vi "NaMCU_configure.vi"() -> ()   [LabVIEW 2016]
uses:
  Instrument drivers/Arduino/ctls_and_globals/Arduino tx msg cluster.ctl
panel:
  in  "DIO 1 mode":u8(ring)=1 items=["Input", "Output"]
  in  "DIO 0 mode":u8(ring)=1 items=["Input", "Output"]
  in  "T1 offset (deg C)":dbl
  in  "T0 offset (deg C)":dbl
  in  "P_atmos offset (Pa)":dbl
  in  "Port":refnum<visa-resource-name>
  in  "Get / Set":u8(ring) items=["Get", "Set"]
  in  "Apply pressure corrections":bool=TRUE
  in  "Tube_D (mm)":dbl=1.0
  in  "Tube_L (mm)":dbl
  out "Read-back":string
  in  "dP offset (Pa)":dbl
  out "Status comment":string
  in  "Address":u8=1
  # "Use this vi to configure the NaMCU pressure transducer node\nThese settings are retained in EEPROM and recalled on power-up."
  # "PN 17/01/2017"
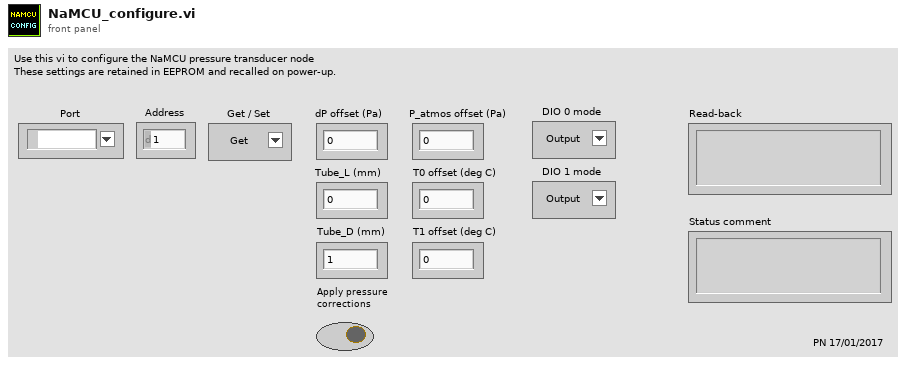
[diagram p1: front panel]
types:
  T1 = typedef "Arduino tx msg cluster.ctl" = cluster{"dest":u8, "A/D/C/I":string, "R/W":string, "chan":u8, "val (float)":sgl}
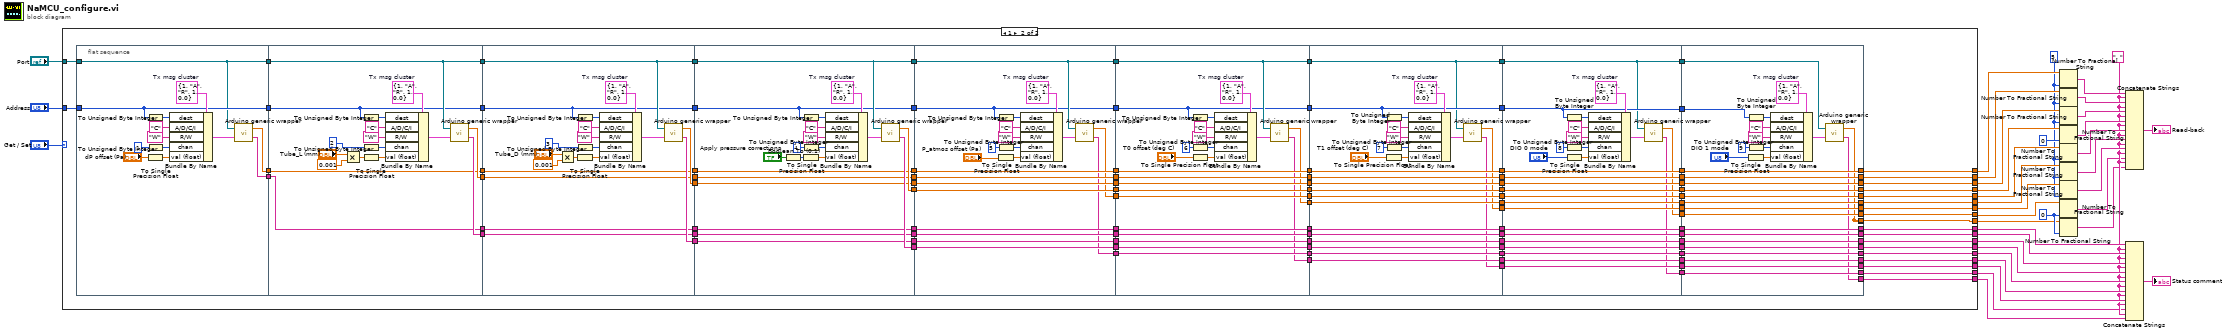
[diagram p0: block diagram]
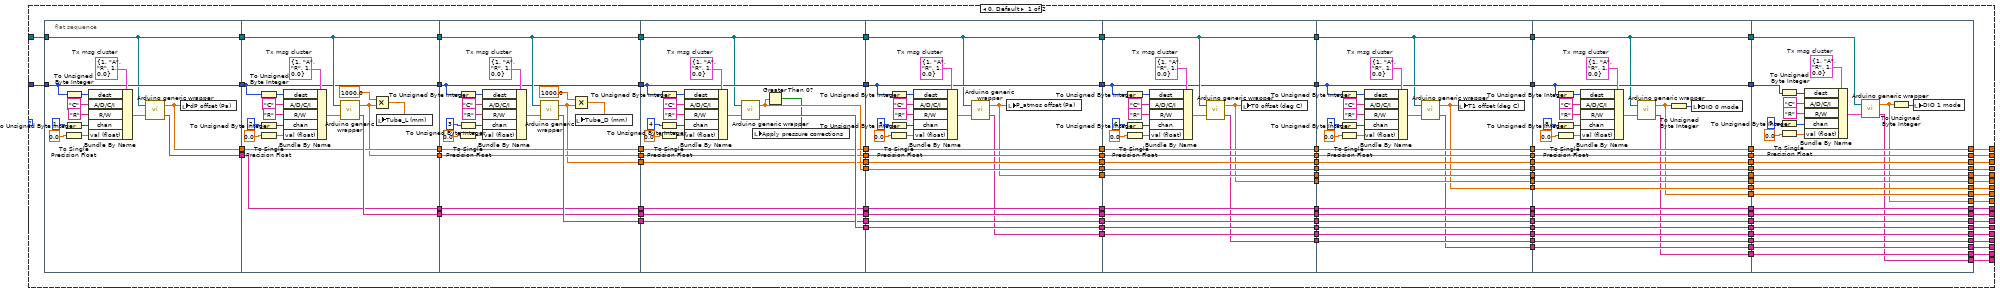
[diagram p2: hidden frame]
diagram:
  w8 = i16 0 ("precision (6)")
  w9 = i16 5 ("precision (6)")
  w7 = ", "
  n1 = case shown="1" "Get / Set" {
    tunnel: "Address" -> [w125 w430]
    tunnel: [w117 w429] -> w31
    tunnel: [w121 w428] -> w30
    tunnel: [w122 w427] -> w28
    tunnel: [w118 w426] -> w27
    tunnel: [w119 w425] -> w26
    tunnel: [w120 w424] -> w25
    tunnel: [w123 w423] -> w24
    tunnel: [w124 w422] -> w23
    tunnel: "Port" -> [w126 w421]
    tunnel: [w84 w410] -> w15
    tunnel: [w78 w396] -> w14
    tunnel: [w75 w380] -> w13
    tunnel: [w82 w409] -> w12
    tunnel: [w79 w395] -> w11
    tunnel: [w76 w379] -> w10
    tunnel: [w43 w347] -> w4
    tunnel: [w42 w345] -> w3
    tunnel: [w38 w342] -> w2
    tunnel: [w37 w341] -> w1
    frame 0, Default {
      n2 = flat-sequence {
        tunnel: w125 -> [w149]
        tunnel: w126 -> [w148]
        tunnel: [w148] -> w144
        tunnel: [w149] -> w143
        tunnel: [w145] -> w142
        tunnel: [w147] -> w141
        tunnel: [w166] -> w140
        tunnel: [w165] -> w139
        tunnel: [w164] -> w138
        tunnel: [w159] -> w137
        tunnel: w144 -> [w166]
        tunnel: w143 -> [w165]
        tunnel: w142 -> [w162]
        tunnel: w141 -> [w163]
        tunnel: [w163] -> w136
        tunnel: [w162] -> w135
        tunnel: w140 -> [w185]
        tunnel: [w185] -> w134
        tunnel: w139 -> [w184]
        tunnel: [w184] -> w133
        tunnel: w138 -> [w182]
        tunnel: w137 -> [w180]
        tunnel: [w183] -> w132
        tunnel: [w176] -> w131
        tunnel: [w182] -> w130
        tunnel: [w181] -> w129
        tunnel: w136 -> [w181]
        tunnel: [w180] -> w128
        tunnel: [w179] -> w127
        tunnel: w135 -> [w179]
        tunnel: w134 -> [w194]
        tunnel: w133 -> [w195]
        tunnel: w132 -> [w203]
        tunnel: w131 -> [w204]
        tunnel: w130 -> [w202]
        tunnel: w129 -> [w201]
        tunnel: w128 -> [w200]
        tunnel: w127 -> [w199]
        tunnel: [w205] -> w116
        tunnel: [w197] -> w115
        tunnel: [w204] -> w114
        tunnel: [w203] -> w113
        tunnel: [w202] -> w112
        tunnel: [w201] -> w111
        tunnel: [w200] -> w110
        tunnel: [w199] -> w109
        tunnel: [w195] -> w92
        tunnel: [w194] -> w91
        tunnel: w116 -> [w234]
        tunnel: w115 -> [w233]
        tunnel: w114 -> [w232]
        tunnel: w113 -> [w231]
        tunnel: w112 -> [w230]
        tunnel: w111 -> [w229]
        tunnel: w110 -> [w228]
        tunnel: w109 -> [w227]
        tunnel: [w234] -> w108
        tunnel: [w233] -> w107
        tunnel: [w232] -> w106
        tunnel: [w231] -> w105
        tunnel: [w230] -> w104
        tunnel: [w229] -> w103
        tunnel: [w228] -> w102
        tunnel: [w227] -> w101
        tunnel: w92 -> [w217]
        tunnel: w91 -> [w216]
        tunnel: [w217] -> w90
        tunnel: [w216] -> w89
        tunnel: [w215] -> w86
        tunnel: [w214] -> w85
        tunnel: w108 -> [w257]
        tunnel: w107 -> [w256]
        tunnel: w106 -> [w255]
        tunnel: w105 -> [w254]
        tunnel: w104 -> [w253]
        tunnel: w103 -> [w252]
        tunnel: w102 -> [w251]
        tunnel: w101 -> [w250]
        tunnel: [w257] -> w100
        tunnel: [w256] -> w99
        tunnel: [w255] -> w98
        tunnel: [w254] -> w97
        tunnel: [w253] -> w96
        tunnel: [w252] -> w95
        tunnel: [w251] -> w94
        tunnel: [w250] -> w93
        tunnel: w90 -> [w237]
        tunnel: w89 -> [w238]
        tunnel: [w237] -> w88
        tunnel: [w238] -> w87
        tunnel: w86 -> [w249]
        tunnel: w85 -> [w248]
        tunnel: [w249] -> w83
        tunnel: [w248] -> w81
        tunnel: [w236] -> w80
        tunnel: [w235] -> w77
        tunnel: w100 -> [w282]
        tunnel: w99 -> [w281]
        tunnel: w98 -> [w280]
        tunnel: w97 -> [w279]
        tunnel: w96 -> [w278]
        tunnel: w95 -> [w277]
        tunnel: w94 -> [w276]
        tunnel: w93 -> [w275]
        tunnel: w88 -> [w259]
        tunnel: w87 -> [w258]
        tunnel: w83 -> [w274]
        tunnel: w81 -> [w273]
        tunnel: w80 -> [w272]
        tunnel: w77 -> [w271]
        tunnel: [w282] -> w74
        tunnel: [w281] -> w73
        tunnel: [w280] -> w72
        tunnel: [w279] -> w71
        tunnel: [w278] -> w70
        tunnel: [w277] -> w69
        tunnel: [w276] -> w68
        tunnel: [w275] -> w67
        tunnel: [w274] -> w66
        tunnel: [w273] -> w65
        tunnel: [w272] -> w64
        tunnel: [w271] -> w63
        tunnel: [w261] -> w62
        tunnel: [w260] -> w61
        tunnel: [w259] -> w46
        tunnel: [w258] -> w45
        tunnel: w74 -> [w310]
        tunnel: w73 -> [w309]
        tunnel: w72 -> [w308]
        tunnel: w71 -> [w307]
        tunnel: w70 -> [w306]
        tunnel: w69 -> [w305]
        tunnel: w68 -> [w304]
        tunnel: w67 -> [w303]
        tunnel: w66 -> [w302]
        tunnel: w65 -> [w301]
        tunnel: w64 -> [w300]
        tunnel: w63 -> [w299]
        tunnel: w62 -> [w298]
        tunnel: w61 -> [w297]
        tunnel: [w310] -> w60
        tunnel: [w309] -> w59
        tunnel: [w308] -> w58
        tunnel: [w307] -> w57
        tunnel: [w306] -> w56
        tunnel: [w305] -> w55
        tunnel: [w304] -> w54
        tunnel: [w303] -> w53
        tunnel: [w302] -> w52
        tunnel: [w301] -> w51
        tunnel: [w300] -> w50
        tunnel: [w299] -> w49
        tunnel: [w298] -> w48
        tunnel: [w297] -> w47
        tunnel: w46 -> [w284]
        tunnel: w45 -> [w283]
        tunnel: [w286] -> w44
        tunnel: [w285] -> w41
        tunnel: [w284] -> w40
        tunnel: [w283] -> w39
        tunnel: [w327] -> w75
        tunnel: [w328] -> w76
        tunnel: [w329] -> w78
        tunnel: [w330] -> w79
        tunnel: [w331] -> w82
        tunnel: [w332] -> w84
        tunnel: [w333] -> w124
        tunnel: [w334] -> w123
        tunnel: [w335] -> w120
        tunnel: [w336] -> w119
        tunnel: [w337] -> w118
        tunnel: [w338] -> w122
        tunnel: [w339] -> w121
        tunnel: [w340] -> w117
        tunnel: w60 -> [w340]
        tunnel: w59 -> [w339]
        tunnel: w58 -> [w338]
        tunnel: w57 -> [w337]
        tunnel: w56 -> [w336]
        tunnel: w55 -> [w335]
        tunnel: w54 -> [w334]
        tunnel: w53 -> [w333]
        tunnel: w52 -> [w332]
        tunnel: w51 -> [w331]
        tunnel: w50 -> [w330]
        tunnel: w49 -> [w329]
        tunnel: w48 -> [w328]
        tunnel: w47 -> [w327]
        tunnel: w44 -> [w326]
        tunnel: [w326] -> w43
        tunnel: [w325] -> w42
        tunnel: w41 -> [w325]
        tunnel: w40 -> [w315]
        tunnel: w39 -> [w314]
        tunnel: [w312] -> w38
        tunnel: [w311] -> w37
        frame #0 {
          w157 = T1 {"dest"=1, "A/D/C/I"="A", "R/W"="R", "chan"=1, "val (float)"=0.0}  # Tx msg cluster
          n3 = To Unsigned Byte Integer(number=w149) -> (unsigned 8bit integer=w155:u8)
          n4 = To Unsigned Byte Integer(number=u8 1) -> (unsigned 8bit integer=w156:u8)
          n5 = To Single Precision Float(number=0.0) -> (single precision float=w153:sgl)
          n6 = Bundle By Name(cluster=w157, "dest"=w155, "A/D/C/I"="C" ("A/D"), "R/W"="R", "chan"=w156, "val (float)"=w153) -> (w154:T1)
          n7 = call "Arduino generic wrapper.vi"("Tx msg cluster"=w154, "Port name"=w148) -> ("Scan comment"=w147:string, "Output"=w145:dbl)
          n8 = local write "dP offset (Pa)"(w145) -> ()
        }
        frame #1 {
          w167 = T1 {"dest"=1, "A/D/C/I"="A", "R/W"="R", "chan"=1, "val (float)"=0.0}  # Tx msg cluster
          n9 = To Unsigned Byte Integer(number=w165) -> (unsigned 8bit integer=w169:u8)
          n10 = To Unsigned Byte Integer(number=u8 2) -> (unsigned 8bit integer=w168:u8)
          n11 = To Single Precision Float(number=0.0) -> (single precision float=w171:sgl)
          n12 = Bundle By Name(cluster=w167, "dest"=w169, "A/D/C/I"="C" ("A/D"), "R/W"="R", "chan"=w168, "val (float)"=w171) -> (w170:T1)
          n13 = call "Arduino generic wrapper.vi"("Tx msg cluster"=w170, "Port name"=w166) -> ("Scan comment"=w164:string, "Output"=w159:dbl)
          n14 = Multiply(x=1000.0 ("y"), y=w159) -> (x*y=w158:dbl)
          n15 = local write "Tube_L (mm)"(w158) -> ()
        }
        frame #2 {
          w193 = T1 {"dest"=1, "A/D/C/I"="A", "R/W"="R", "chan"=1, "val (float)"=0.0}  # Tx msg cluster
          n16 = To Unsigned Byte Integer(number=w184) -> (unsigned 8bit integer=w191:u8)
          n17 = To Unsigned Byte Integer(number=u8 3) -> (unsigned 8bit integer=w192:u8)
          n18 = To Single Precision Float(number=0.0) -> (single precision float=w189:sgl)
          n19 = Bundle By Name(cluster=w193, "dest"=w191, "A/D/C/I"="C" ("A/D"), "R/W"="R", "chan"=w192, "val (float)"=w189) -> (w190:T1)
          n20 = call "Arduino generic wrapper.vi"("Tx msg cluster"=w190, "Port name"=w185) -> ("Scan comment"=w183:string, "Output"=w176:dbl)
          n21 = Multiply(x=1000.0 ("y"), y=w176) -> (x*y=w175:dbl)
          n22 = local write "Tube_D (mm)"(w175) -> ()
        }
        frame #3 {
          w212 = T1 {"dest"=1, "A/D/C/I"="A", "R/W"="R", "chan"=1, "val (float)"=0.0}  # Tx msg cluster
          n23 = To Unsigned Byte Integer(number=w195) -> (unsigned 8bit integer=w206:u8)
          n24 = To Unsigned Byte Integer(number=u8 4) -> (unsigned 8bit integer=w207:u8)
          n25 = To Single Precision Float(number=0.0) -> (single precision float=w209:sgl)
          n26 = Bundle By Name(cluster=w212, "dest"=w206, "A/D/C/I"="C" ("A/D"), "R/W"="R", "chan"=w207, "val (float)"=w209) -> (w208:T1)
          n27 = call "Arduino generic wrapper.vi"("Tx msg cluster"=w208, "Port name"=w194) -> ("Scan comment"=w205:string, "Output"=w197:dbl)
          n28 = Greater Than 0?(x=w197) -> (x > 0?=w196:bool)
          n29 = local write "Apply pressure corrections"(w196) -> ()
        }
        frame #4 {
          w219 = T1 {"dest"=1, "A/D/C/I"="A", "R/W"="R", "chan"=1, "val (float)"=0.0}  # Tx msg cluster
          n30 = To Unsigned Byte Integer(number=w217) -> (unsigned 8bit integer=w225:u8)
          n31 = To Unsigned Byte Integer(number=u8 5) -> (unsigned 8bit integer=w224:u8)
          n32 = To Single Precision Float(number=0.0) -> (single precision float=w222:sgl)
          n33 = Bundle By Name(cluster=w219, "dest"=w225, "A/D/C/I"="C" ("A/D"), "R/W"="R", "chan"=w224, "val (float)"=w222) -> (w223:T1)
          n34 = call "Arduino generic wrapper.vi"("Tx msg cluster"=w223, "Port name"=w216) -> ("Scan comment"=w215:string, "Output"=w214:dbl)
          n35 = local write "P_atmos offset (Pa)"(w214) -> ()
        }
        frame #5 {
          w246 = T1 {"dest"=1, "A/D/C/I"="A", "R/W"="R", "chan"=1, "val (float)"=0.0}  # Tx msg cluster
          n36 = To Unsigned Byte Integer(number=w237) -> (unsigned 8bit integer=w240:u8)
          n37 = To Unsigned Byte Integer(number=u8 6) -> (unsigned 8bit integer=w241:u8)
          n38 = To Single Precision Float(number=0.0) -> (single precision float=w243:sgl)
          n39 = Bundle By Name(cluster=w246, "dest"=w240, "A/D/C/I"="C" ("A/D"), "R/W"="R", "chan"=w241, "val (float)"=w243) -> (w242:T1)
          n40 = call "Arduino generic wrapper.vi"("Tx msg cluster"=w242, "Port name"=w238) -> ("Scan comment"=w235:string, "Output"=w236:dbl)
          n41 = local write "T0 offset (deg C)"(w236) -> ()
        }
        frame #6 {
          w263 = T1 {"dest"=1, "A/D/C/I"="A", "R/W"="R", "chan"=1, "val (float)"=0.0}  # Tx msg cluster
          n42 = To Unsigned Byte Integer(number=w259) -> (unsigned 8bit integer=w269:u8)
          n43 = To Unsigned Byte Integer(number=u8 7) -> (unsigned 8bit integer=w268:u8)
          n44 = To Single Precision Float(number=0.0) -> (single precision float=w266:sgl)
          n45 = Bundle By Name(cluster=w263, "dest"=w269, "A/D/C/I"="C" ("A/D"), "R/W"="R", "chan"=w268, "val (float)"=w266) -> (w267:T1)
          n46 = call "Arduino generic wrapper.vi"("Tx msg cluster"=w267, "Port name"=w258) -> ("Scan comment"=w260:string, "Output"=w261:dbl)
          n47 = local write "T1 offset (deg C)"(w261) -> ()
        }
        frame #7 {
          w295 = T1 {"dest"=1, "A/D/C/I"="A", "R/W"="R", "chan"=1, "val (float)"=0.0}  # Tx msg cluster
          n48 = To Unsigned Byte Integer(number=w284) -> (unsigned 8bit integer=w289:u8)
          n49 = To Unsigned Byte Integer(number=u8 8) -> (unsigned 8bit integer=w290:u8)
          n50 = To Single Precision Float(number=0.0) -> (single precision float=w292:sgl)
          n51 = Bundle By Name(cluster=w295, "dest"=w289, "A/D/C/I"="C" ("A/D"), "R/W"="R", "chan"=w290, "val (float)"=w292) -> (w291:T1)
          n52 = call "Arduino generic wrapper.vi"("Tx msg cluster"=w291, "Port name"=w283) -> ("Scan comment"=w286:string, "Output"=w285:dbl)
          n53 = To Unsigned Byte Integer(number=w285) -> (unsigned 8bit integer=w287:u8)
          n54 = local write "DIO 0 mode"(w287) -> ()
        }
        frame #8 {
          w317 = T1 {"dest"=1, "A/D/C/I"="A", "R/W"="R", "chan"=1, "val (float)"=0.0}  # Tx msg cluster
          n55 = To Unsigned Byte Integer(number=w315) -> (unsigned 8bit integer=w323:u8)
          n56 = To Unsigned Byte Integer(number=u8 9) -> (unsigned 8bit integer=w322:u8)
          n57 = To Single Precision Float(number=0.0) -> (single precision float=w320:sgl)
          n58 = Bundle By Name(cluster=w317, "dest"=w323, "A/D/C/I"="C" ("A/D"), "R/W"="R", "chan"=w322, "val (float)"=w320) -> (w321:T1)
          n59 = call "Arduino generic wrapper.vi"("Tx msg cluster"=w321, "Port name"=w314) -> ("Scan comment"=w312:string, "Output"=w311:dbl)
          n60 = To Unsigned Byte Integer(number=w311) -> (unsigned 8bit integer=w313:u8)
          n61 = local write "DIO 1 mode"(w313) -> ()
        }
      }
    }
    frame 1 {
      n62 = flat-sequence {
        tunnel: w430 -> [w453]
        tunnel: w421 -> [w452]
        tunnel: [w452] -> w448
        tunnel: [w453] -> w447
        tunnel: [w451] -> w446
        tunnel: [w450] -> w445
        tunnel: [w470] -> w444
        tunnel: [w469] -> w443
        tunnel: [w468] -> w442
        tunnel: [w467] -> w441
        tunnel: w448 -> [w470]
        tunnel: w447 -> [w469]
        tunnel: w446 -> [w465]
        tunnel: w445 -> [w466]
        tunnel: [w466] -> w440
        tunnel: [w465] -> w439
        tunnel: w444 -> [w489]
        tunnel: [w489] -> w438
        tunnel: w443 -> [w488]
        tunnel: [w488] -> w437
        tunnel: w442 -> [w485]
        tunnel: w441 -> [w483]
        tunnel: [w487] -> w436
        tunnel: [w486] -> w435
        tunnel: [w485] -> w434
        tunnel: [w484] -> w433
        tunnel: w440 -> [w484]
        tunnel: [w483] -> w432
        tunnel: [w482] -> w431
        tunnel: w439 -> [w482]
        tunnel: w438 -> [w499]
        tunnel: w437 -> [w498]
        tunnel: w436 -> [w504]
        tunnel: w435 -> [w505]
        tunnel: w434 -> [w503]
        tunnel: w433 -> [w502]
        tunnel: w432 -> [w501]
        tunnel: w431 -> [w500]
        tunnel: [w509] -> w420
        tunnel: [w508] -> w419
        tunnel: [w505] -> w418
        tunnel: [w504] -> w417
        tunnel: [w503] -> w416
        tunnel: [w502] -> w415
        tunnel: [w501] -> w414
        tunnel: [w500] -> w413
        tunnel: [w499] -> w412
        tunnel: [w498] -> w411
        tunnel: w420 -> [w538]
        tunnel: w419 -> [w537]
        tunnel: w418 -> [w536]
        tunnel: w417 -> [w535]
        tunnel: w416 -> [w534]
        tunnel: w415 -> [w533]
        tunnel: w414 -> [w532]
        tunnel: w413 -> [w531]
        tunnel: w412 -> [w519]
        tunnel: w411 -> [w518]
        tunnel: [w538] -> w408
        tunnel: [w537] -> w407
        tunnel: [w536] -> w406
        tunnel: [w535] -> w405
        tunnel: [w534] -> w404
        tunnel: [w533] -> w403
        tunnel: [w532] -> w402
        tunnel: [w531] -> w401
        tunnel: [w521] -> w400
        tunnel: [w520] -> w399
        tunnel: [w519] -> w398
        tunnel: [w518] -> w397
        tunnel: w408 -> [w561]
        tunnel: w407 -> [w560]
        tunnel: w406 -> [w559]
        tunnel: w405 -> [w558]
        tunnel: w404 -> [w557]
        tunnel: w403 -> [w556]
        tunnel: w402 -> [w555]
        tunnel: w401 -> [w554]
        tunnel: w400 -> [w553]
        tunnel: w399 -> [w552]
        tunnel: w398 -> [w540]
        tunnel: w397 -> [w539]
        tunnel: [w561] -> w394
        tunnel: [w560] -> w393
        tunnel: [w559] -> w392
        tunnel: [w558] -> w391
        tunnel: [w557] -> w390
        tunnel: [w556] -> w389
        tunnel: [w555] -> w388
        tunnel: [w554] -> w387
        tunnel: [w553] -> w386
        tunnel: [w552] -> w385
        tunnel: [w542] -> w384
        tunnel: [w541] -> w383
        tunnel: [w540] -> w382
        tunnel: [w539] -> w381
        tunnel: w394 -> [w586]
        tunnel: w393 -> [w585]
        tunnel: w392 -> [w584]
        tunnel: w391 -> [w583]
        tunnel: w390 -> [w582]
        tunnel: w389 -> [w581]
        tunnel: w388 -> [w580]
        tunnel: w387 -> [w579]
        tunnel: w386 -> [w578]
        tunnel: w385 -> [w577]
        tunnel: w384 -> [w576]
        tunnel: w383 -> [w575]
        tunnel: w382 -> [w562]
        tunnel: w381 -> [w563]
        tunnel: [w586] -> w378
        tunnel: [w585] -> w377
        tunnel: [w584] -> w376
        tunnel: [w583] -> w375
        tunnel: [w582] -> w374
        tunnel: [w581] -> w373
        tunnel: [w580] -> w372
        tunnel: [w579] -> w371
        tunnel: [w578] -> w370
        tunnel: [w577] -> w369
        tunnel: [w576] -> w368
        tunnel: [w575] -> w367
        tunnel: [w565] -> w366
        tunnel: [w564] -> w365
        tunnel: [w563] -> w350
        tunnel: [w562] -> w349
        tunnel: w378 -> [w613]
        tunnel: w377 -> [w612]
        tunnel: w376 -> [w611]
        tunnel: w375 -> [w610]
        tunnel: w374 -> [w609]
        tunnel: w373 -> [w608]
        tunnel: w372 -> [w607]
        tunnel: w371 -> [w606]
        tunnel: w370 -> [w605]
        tunnel: w369 -> [w604]
        tunnel: w368 -> [w603]
        tunnel: w367 -> [w602]
        tunnel: w366 -> [w601]
        tunnel: w365 -> [w600]
        tunnel: [w613] -> w364
        tunnel: [w612] -> w363
        tunnel: [w611] -> w362
        tunnel: [w610] -> w361
        tunnel: [w609] -> w360
        tunnel: [w608] -> w359
        tunnel: [w607] -> w358
        tunnel: [w606] -> w357
        tunnel: [w605] -> w356
        tunnel: [w604] -> w355
        tunnel: [w603] -> w354
        tunnel: [w602] -> w353
        tunnel: [w601] -> w352
        tunnel: [w600] -> w351
        tunnel: w350 -> [w588]
        tunnel: w349 -> [w587]
        tunnel: [w590] -> w348
        tunnel: [w589] -> w346
        tunnel: [w588] -> w344
        tunnel: [w587] -> w343
        tunnel: [w629] -> w379
        tunnel: [w630] -> w380
        tunnel: [w631] -> w395
        tunnel: [w632] -> w396
        tunnel: [w633] -> w409
        tunnel: [w634] -> w410
        tunnel: [w635] -> w422
        tunnel: [w636] -> w423
        tunnel: [w637] -> w424
        tunnel: [w638] -> w425
        tunnel: [w639] -> w426
        tunnel: [w640] -> w427
        tunnel: [w641] -> w428
        tunnel: [w642] -> w429
        tunnel: w364 -> [w642]
        tunnel: w363 -> [w641]
        tunnel: w362 -> [w640]
        tunnel: w361 -> [w639]
        tunnel: w360 -> [w638]
        tunnel: w359 -> [w637]
        tunnel: w358 -> [w636]
        tunnel: w357 -> [w635]
        tunnel: w356 -> [w634]
        tunnel: w355 -> [w633]
        tunnel: w354 -> [w632]
        tunnel: w353 -> [w631]
        tunnel: w352 -> [w630]
        tunnel: w351 -> [w629]
        tunnel: w348 -> [w628]
        tunnel: [w628] -> w347
        tunnel: w346 -> [w627]
        tunnel: [w627] -> w345
        tunnel: w344 -> [w618]
        tunnel: w343 -> [w617]
        tunnel: [w615] -> w342
        tunnel: [w614] -> _
        tunnel: [w614] -> w341
        frame #0 {
          w461 = T1 {"dest"=1, "A/D/C/I"="A", "R/W"="R", "chan"=1, "val (float)"=0.0}  # Tx msg cluster
          n63 = To Unsigned Byte Integer(number=w453) -> (unsigned 8bit integer=w459:u8)
          n64 = To Unsigned Byte Integer(number=u8 1) -> (unsigned 8bit integer=w460:u8)
          n65 = To Single Precision Float(number="dP offset (Pa)") -> (single precision float=w457:sgl)
          n66 = Bundle By Name(cluster=w461, "dest"=w459, "A/D/C/I"="C" ("A/D"), "R/W"="W", "chan"=w460, "val (float)"=w457) -> (w458:T1)
          n67 = call "Arduino generic wrapper.vi"("Tx msg cluster"=w458, "Port name"=w452) -> ("Scan comment"=w450:string, "Output"=w451:dbl)
        }
        frame #1 {
          w471 = T1 {"dest"=1, "A/D/C/I"="A", "R/W"="R", "chan"=1, "val (float)"=0.0}  # Tx msg cluster
          n68 = Multiply(x="Tube_L (mm)", y=0.001) -> (x*y=w463:dbl)
          n69 = To Unsigned Byte Integer(number=w469) -> (unsigned 8bit integer=w473:u8)
          n70 = To Unsigned Byte Integer(number=u8 2) -> (unsigned 8bit integer=w472:u8)
          n71 = To Single Precision Float(number=w463) -> (single precision float=w475:sgl)
          n72 = Bundle By Name(cluster=w471, "dest"=w473, "A/D/C/I"="C" ("A/D"), "R/W"="W", "chan"=w472, "val (float)"=w475) -> (w474:T1)
          n73 = call "Arduino generic wrapper.vi"("Tx msg cluster"=w474, "Port name"=w470) -> ("Scan comment"=w468:string, "Output"=w467:dbl)
        }
        frame #2 {
          w497 = T1 {"dest"=1, "A/D/C/I"="A", "R/W"="R", "chan"=1, "val (float)"=0.0}  # Tx msg cluster
          n74 = Multiply(x="Tube_D (mm)", y=0.001) -> (x*y=w479:dbl)
          n75 = To Unsigned Byte Integer(number=w488) -> (unsigned 8bit integer=w495:u8)
          n76 = To Unsigned Byte Integer(number=u8 3) -> (unsigned 8bit integer=w496:u8)
          n77 = To Single Precision Float(number=w479) -> (single precision float=w493:sgl)
          n78 = Bundle By Name(cluster=w497, "dest"=w495, "A/D/C/I"="C" ("A/D"), "R/W"="W", "chan"=w496, "val (float)"=w493) -> (w494:T1)
          n79 = call "Arduino generic wrapper.vi"("Tx msg cluster"=w494, "Port name"=w489) -> ("Scan comment"=w487:string, "Output"=w486:dbl)
        }
        frame #3 {
          w516 = T1 {"dest"=1, "A/D/C/I"="A", "R/W"="R", "chan"=1, "val (float)"=0.0}  # Tx msg cluster
          n80 = Boolean To (0,1)(Boolean="Apply pressure corrections") -> (0, 1=w506:i16)
          n81 = To Unsigned Byte Integer(number=w498) -> (unsigned 8bit integer=w510:u8)
          n82 = To Unsigned Byte Integer(number=u8 4) -> (unsigned 8bit integer=w511:u8)
          n83 = To Single Precision Float(number=w506) -> (single precision float=w513:sgl)
          n84 = Bundle By Name(cluster=w516, "dest"=w510, "A/D/C/I"="C" ("A/D"), "R/W"="W", "chan"=w511, "val (float)"=w513) -> (w512:T1)
          n85 = call "Arduino generic wrapper.vi"("Tx msg cluster"=w512, "Port name"=w499) -> ("Scan comment"=w509:string, "Output"=w508:dbl)
        }
        frame #4 {
          w524 = T1 {"dest"=1, "A/D/C/I"="A", "R/W"="R", "chan"=1, "val (float)"=0.0}  # Tx msg cluster
          n86 = To Unsigned Byte Integer(number=w518) -> (unsigned 8bit integer=w530:u8)
          n87 = To Unsigned Byte Integer(number=u8 5) -> (unsigned 8bit integer=w529:u8)
          n88 = To Single Precision Float(number="P_atmos offset (Pa)") -> (single precision float=w527:sgl)
          n89 = Bundle By Name(cluster=w524, "dest"=w530, "A/D/C/I"="C" ("A/D"), "R/W"="W", "chan"=w529, "val (float)"=w527) -> (w528:T1)
          n90 = call "Arduino generic wrapper.vi"("Tx msg cluster"=w528, "Port name"=w519) -> ("Scan comment"=w521:string, "Output"=w520:dbl)
        }
        frame #5 {
          w550 = T1 {"dest"=1, "A/D/C/I"="A", "R/W"="R", "chan"=1, "val (float)"=0.0}  # Tx msg cluster
          n91 = To Unsigned Byte Integer(number=w539) -> (unsigned 8bit integer=w544:u8)
          n92 = To Unsigned Byte Integer(number=u8 6) -> (unsigned 8bit integer=w545:u8)
          n93 = To Single Precision Float(number="T0 offset (deg C)") -> (single precision float=w547:sgl)
          n94 = Bundle By Name(cluster=w550, "dest"=w544, "A/D/C/I"="C" ("A/D"), "R/W"="W", "chan"=w545, "val (float)"=w547) -> (w546:T1)
          n95 = call "Arduino generic wrapper.vi"("Tx msg cluster"=w546, "Port name"=w540) -> ("Scan comment"=w542:string, "Output"=w541:dbl)
        }
        frame #6 {
          w568 = T1 {"dest"=1, "A/D/C/I"="A", "R/W"="R", "chan"=1, "val (float)"=0.0}  # Tx msg cluster
          n96 = To Unsigned Byte Integer(number=w563) -> (unsigned 8bit integer=w574:u8)
          n97 = To Unsigned Byte Integer(number=u8 7) -> (unsigned 8bit integer=w573:u8)
          n98 = To Single Precision Float(number="T1 offset (deg C)") -> (single precision float=w571:sgl)
          n99 = Bundle By Name(cluster=w568, "dest"=w574, "A/D/C/I"="C" ("A/D"), "R/W"="W", "chan"=w573, "val (float)"=w571) -> (w572:T1)
          n100 = call "Arduino generic wrapper.vi"("Tx msg cluster"=w572, "Port name"=w562) -> ("Scan comment"=w565:string, "Output"=w564:dbl)
        }
        frame #7 {
          w598 = T1 {"dest"=1, "A/D/C/I"="A", "R/W"="R", "chan"=1, "val (float)"=0.0}  # Tx msg cluster
          n101 = To Unsigned Byte Integer(number=w588) -> (unsigned 8bit integer=w592:u8)
          n102 = To Unsigned Byte Integer(number=u8 8) -> (unsigned 8bit integer=w593:u8)
          n103 = To Single Precision Float(number="DIO 0 mode") -> (single precision float=w595:sgl)
          n104 = Bundle By Name(cluster=w598, "dest"=w592, "A/D/C/I"="C" ("A/D"), "R/W"="W", "chan"=w593, "val (float)"=w595) -> (w594:T1)
          n105 = call "Arduino generic wrapper.vi"("Tx msg cluster"=w594, "Port name"=w587) -> ("Scan comment"=w590:string, "Output"=w589:dbl)
        }
        frame #8 {
          w620 = T1 {"dest"=1, "A/D/C/I"="A", "R/W"="R", "chan"=1, "val (float)"=0.0}  # Tx msg cluster
          n106 = To Unsigned Byte Integer(number=w618) -> (unsigned 8bit integer=w626:u8)
          n107 = To Unsigned Byte Integer(number=u8 9) -> (unsigned 8bit integer=w625:u8)
          n108 = To Single Precision Float(number="DIO 1 mode") -> (single precision float=w623:sgl)
          n109 = Bundle By Name(cluster=w620, "dest"=w626, "A/D/C/I"="C" ("A/D"), "R/W"="W", "chan"=w625, "val (float)"=w623) -> (w624:T1)
          n110 = call "Arduino generic wrapper.vi"("Tx msg cluster"=w624, "Port name"=w617) -> ("Scan comment"=w615:string, "Output"=w614:dbl)
        }
      }
    }
  }
  n111 = Number To Fractional String(number=w23, precision (6)=w9) -> (F-format string=w35:string)  [unwired: 2 in]
  n112 = Number To Fractional String(number=w24, precision (6)=w9) -> (F-format string=w34:string)  [unwired: 2 in]
  n113 = Number To Fractional String(number=w28, precision (6)=w9) -> (F-format string=w22:string)  [unwired: 2 in]
  n114 = Number To Fractional String(number=w30, precision (6)=i16 0) -> (F-format string=w21:string)  [unwired: 2 in]
  n115 = Number To Fractional String(number=w12, precision (6)=w9) -> (F-format string=w18:string)  [unwired: 2 in]
  n116 = Number To Fractional String(number=w11, precision (6)=w9) -> (F-format string=w17:string)  [unwired: 2 in]
  n117 = Number To Fractional String(number=w10, precision (6)=w9) -> (F-format string=w16:string)  [unwired: 2 in]
  n118 = Number To Fractional String(number=w3, precision (6)=w8) -> (F-format string=w5:string)  [unwired: 2 in]
  n119 = Number To Fractional String(number=w1, precision (6)=w8) -> (F-format string=w6:string)  [unwired: 2 in]
  n120 = Concatenate Strings(w35, w7, w34, w7, w22, w7, w21, w7, w18, w7, w17, w7, w16, w7, w5, w7, w6) -> (→"Read-back":string)
  n121 = Concatenate Strings(w25, w7, w26, w7, w27, w7, w31, w7, w15, w7, w14, w7, w13, w7, w4, w7, w2) -> (→"Status comment":string)
